vi "Connect String.vi"(8 "Error In":errorcluster, 10 "Signal":string, 11 "Sender In":refnum<class "LQObject.lvclass">) -> (0 "Error Out":errorcluster, 2 "String Signal":refnum<user-event>, 3 "Sender Out":refnum<class "LQObject.lvclass">)   [LabVIEW 2013, in "Template.lvlib" / "LQWidgetEngine.lvclass"]
uses:
  LQWidgetEngine.lvclass
  LQObject/LQObject.lvclass
  LQObject/LQObject.lvclass/LQObject.ctl
  Connection Action.ctl
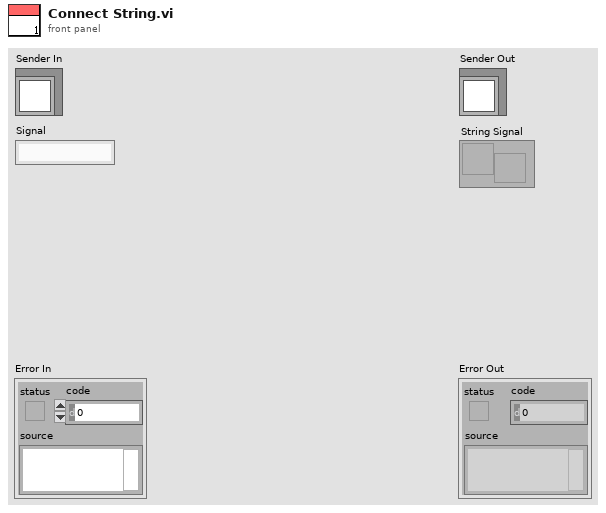
[diagram p1: front panel]
types:
  T1 = typedef "Template.lvlib/LQWidgetEngine.lvclass/Connection Action.ctl" = enum16{"Init", "Add Connection", "Get Connections", "Clean Up"}
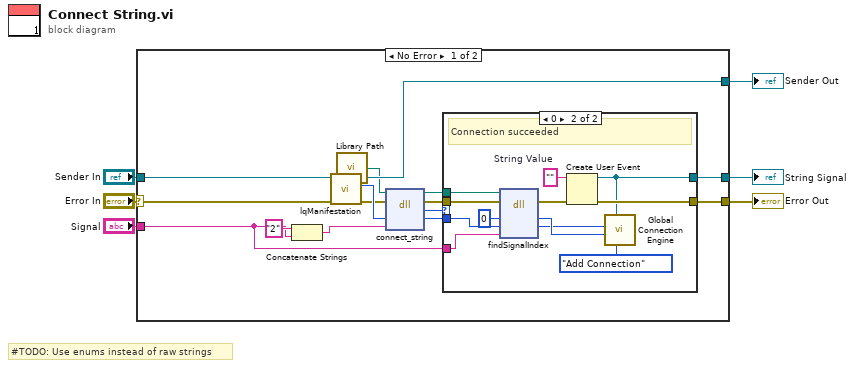
[diagram p0: block diagram]
diagram:
  # "#TODO: Use enums instead of raw strings"
  n1 = case shown="No Error" "Error In" {
    selector: "Error In" -> [w18 w36]
    tunnel: [w15 w36] -> w5
    tunnel: [w20 w35] -> w3
    tunnel: "Sender In" -> [w21 w35]
    tunnel: "Signal" -> [w8 _]
    tunnel: [w14 _] -> w1
    frame No Error {
      n2 = Concatenate Strings("2" ("string"), w8) -> (w9:string)
      n3 = call "lqManifestation.vi"("error in (no error)"=w18, "QObject in"=w21) -> ("error out"=w17:errorcluster, "Manifestation"=w19:u32, "QObject out"=w20:refnum<class "LQObject.lvclass">)  [unwired: 7 in]
      n4 = call "Library Path.vi"() -> ("Library Path"=w7:path)
      n5 = dll-call lib="?" fn="connect_string"(path in=w7, error in=w17, "obj"=w19, "encodedSignal"=w9) -> (path out=w12:path, error out=w16:errorcluster, "errorCode"=w13:i32, "obj"=w11:u32)  [unwired: 2 in]
      n6 = case shown="0" w13 {
        tunnel: w16 -> [w22 w32]
        tunnel: [w22 w34] -> w15
        tunnel: [_ w25] -> w14
        tunnel: w12 -> [_ w30]
        tunnel: w11 -> [_ w29]
        tunnel: w8 -> [_ w23]
        frame Default {
          # "#TODO: Create error cluster"
          # "Connection failed"
        }
        frame 0 {
          w33 = ""  # String Value
          # "Connection succeeded"
          n7 = dll-call lib="?" fn="findSignalIndex"(path in=w30, error in=w32, "retVal"=i64 0, "obj"=w29, "encodedSignal"=w23) -> (error out=w31:errorcluster, "retVal"=w27:i64, "obj"=w26:u32)  [unwired: 3 in, 1 out]
          n8 = Create User Event(user event datatype=w33, error in=w31) -> (user event=w25:refnum<user-event>, error out=w34:errorcluster)
          n9 = call "Global Connection Engine.vi"("Connection Action"=Connection_Action."Add Connection", "Signal Channel"=w25, "Signal Index"=w27, "QObject Refnum"=w26) -> ()  [unwired: 7 in, 1 out]
        }
      }
    }
    frame Error {
    }
  }
  "Error Out" <- w5
  "Sender Out" <- w3
  "String Signal" <- w1
